vi "Head Graphic.vi"(10 "Stop":bool, 11 "Oculus Data in":T1) -> ()   [LabVIEW 2017]
panel:
  out "Yaw":dbl
  out "Pitch":dbl
  out "Roll":dbl
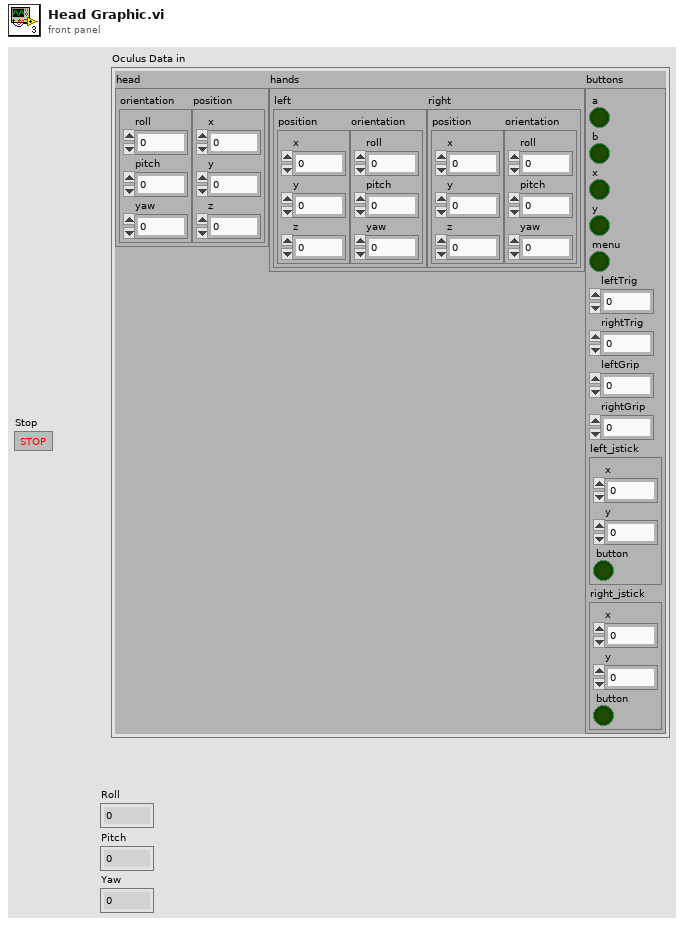
[diagram p1: front panel]
types:
  T1 = cluster{"head":cluster{"orientation":cluster{"roll":dbl, "pitch":dbl, "yaw":dbl}, "position":cluster{"x":dbl, "y":dbl, "z":dbl}}, "hands":cluster{"left":cluster{"position":cluster{"x":dbl, "y":dbl, "z":dbl}, "orientation":cluster{"roll":dbl, "pitch":dbl, "yaw":dbl}}, "right":cluster{"position":cluster{"x":dbl, "y":dbl, "z":dbl}, "orientation":cluster{"roll":dbl, "pitch":dbl, "yaw":dbl}}}, "buttons":cluster{"a":bool, "b":bool, "x":bool, "y":bool, "menu":bool, "leftTrig":dbl, "rightTrig":dbl, "leftGrip":dbl, "rightGrip":dbl, "left_jstick":cluster{"x":dbl, "y":dbl, "button":bool}, "right_jstick":cluster{"x":dbl, "y":dbl, "button":bool}}}
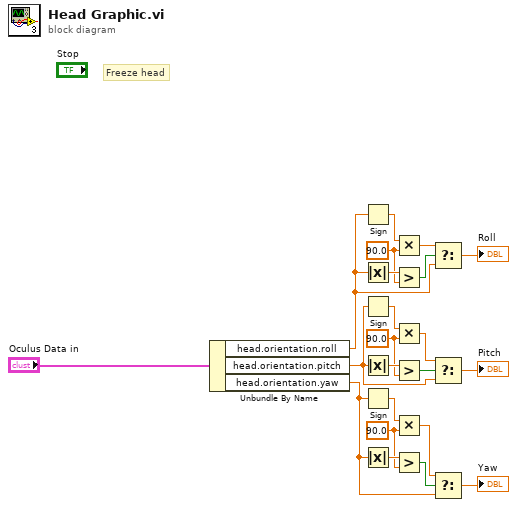
[diagram p0: block diagram]
diagram:
  w7 = 90.0 ("y")
  w12 = 90.0 ("y")
  w17 = 90.0 ("y")
  # "Freeze head"
  n1 = Unbundle By Name("Oculus Data in") -> ("head.orientation.roll"=w19:dbl, "head.orientation.pitch"=w5:dbl, "head.orientation.yaw"=w6:dbl)
  n2 = Sign(1:w19) -> (0:w20:dbl)
  n3 = Absolute Value(x=w19) -> (abs(x)=w22:dbl)
  n4 = Sign(1:w5) -> (0:w14:dbl)
  n5 = Absolute Value(x=w5) -> (abs(x)=w16:dbl)
  n6 = Sign(1:w6) -> (0:w9:dbl)
  n7 = Absolute Value(x=w6) -> (abs(x)=w11:dbl)
  n8 = Multiply(x=w20, y=w17) -> (x*y=w18:dbl)
  n9 = Greater?(x=w22, y=w17) -> (0:w21:bool)
  n10 = Multiply(x=w14, y=w12) -> (x*y=w13:dbl)
  n11 = Greater?(x=w16, y=w12) -> (0:w15:bool)
  n12 = Multiply(x=w9, y=w7) -> (x*y=w8:dbl)
  n13 = Greater?(x=w11, y=w7) -> (0:w10:bool)
  n14 = Select(t=w18, s=w21, f=w19) -> (s? t:f=→"Roll":dbl)
  n15 = Select(t=w13, s=w15, f=w5) -> (s? t:f=→"Pitch":dbl)
  n16 = Select(t=w8, s=w10, f=w6) -> (s? t:f=→"Yaw":dbl)
